vi "Disabled.vi"(7 "Robot Mode":T2, 10 "Match Info":T1={"Autonomous Elapsed Seconds"=0.0, "TeleOp Elapsed Seconds"=0.0, "Disabled Elapsed Seconds"=0.0, "Visited Autonomous"=FALSE, "Visited TeleOp"=FALSE, "Visited Disabled"=FALSE, "Autonomous Settings"={"Autonomous Style"=enum."Independent", "VI Refnum"=refnum}}, 11 "Call Context":T3) -> ()   [LabVIEW 2012]
doc: "This VI is called each time a disabled packet is received from the DS. It is often used to prepare for the next robot mode, to calibrate sensors, etc."
uses:
  <vilib>/Rock Robotics/WPI/DriverStation/WPI_DriverStationDerivedRobotMode.ctl
  <vilib>/Rock Robotics/WPI/DriverStation/WPI_DriverStationRobotMode2.ctl
  <vilib>/Rock Robotics/WPI/DriverStation/WPI_DriverStationMatch Info.ctl
  Robot Global Data.vi
  <vilib>/Rock Robotics/WPI/Joystick/WPI_JoystickGetSetRefNum.vi
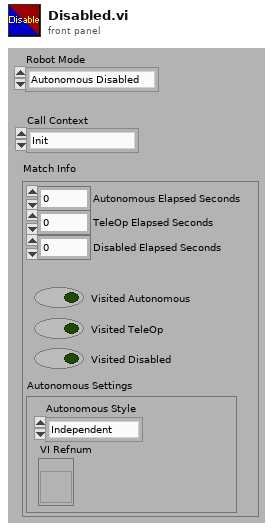
[diagram p1: front panel]
types:
  T1 = typedef "WPI_DriverStationMatch Info.ctl" = cluster{"Autonomous Elapsed Seconds":dbl, "TeleOp Elapsed Seconds":dbl, "Disabled Elapsed Seconds":dbl, "Visited Autonomous":bool, "Visited TeleOp":bool, "Visited Disabled":bool, "Autonomous Settings":cluster{"Autonomous Style":enum16{"Iterative", "Independent"}, "VI Refnum":refnum<vi>}}
  T2 = typedef "WPI_DriverStationRobotMode2.ctl" = enum16{"Autonomous Disabled", "Autonomous Enabled", "Teleop Disabled", "Teleop Enabled", "Timeout", "Finish", "Test Disabled", "Test Enabled"}
  T3 = typedef "WPI_DriverStationDerivedRobotMode.ctl" = enum16{"Init", "Execute", "Stop"}
  T4 = typedef "WPI_JoystickDevRef.ctl" = cluster{"Device":T5}
  T5 = typedef "WPI_JoystickDeviceEnum.ctl" = enum16{"USB 1", "USB 2", "USB 3", "USB 4", "Kinect 1", "Kinect 2"}
  T6 = typedef "WPI_JoystickButtonState.ctl" = cluster{"Button 1":bool, "Button 2":bool, "Button 3":bool, "Button 4":bool, "Button 5":bool, "Button 6":bool, "Button 7":bool, "Button 8":bool, "Button 9":bool, "Button 10":bool, "Button 11":bool, "Button 12":bool}
  T7 = cluster{"FlipperLeftUp":dbl, "FlipperLeftDown":dbl, "FlipperRightUp":dbl, "FlipperRightDown":dbl, "KickerLeftBack":dbl, "KickerLeftForward":dbl, "KickerRightBack":dbl, "KickerRightForward":dbl}
  T8 = typedef "WPI_MotorControlDeviceRef.ctl" = cluster{"DeviceStatus":errorcluster, "Type":enum16{"PWM", "CAN"}, "PWM":cluster{"Digital Module":T9, "PWM Channel":T10, "DeadBand":T11}, "CAN":cluster{"Device Number":u8, "Control Mode":T12, "Semaphore":T13, "Max Vout":dbl}, "Invert":bool, "TransformRef":T14, "InvTransformRef":T14}
  T9 = typedef "FPGA_TypedefDigitalModule.ctl" = enum16{"Digital Module 1", "Digital Module 2"}
  T10 = typedef "FPGA_DIOPWMChannel.ctl" = enum8{"PWM 1", "PWM 2", "PWM 3", "PWM 4", "PWM 5", "PWM 6", "PWM 7", "PWM 8", "PWM 9", "PWM 10", "Invalid"}
  T11 = typedef "WPI_PWMDeadband.ctl" = cluster{"Name":string, "maxPositivePwm":i32, "minPositivePwm":i32, "centerPwm":i32, "maxNegativePwm":i32, "minNegativePwm":i32, "angularRange":u16}
  T12 = typedef "WPI_CANJaguar_ControlMode.ctl" = enum8{"Percent VBus", "Current", "Speed", "Position", "Voltage"}
  T13 = typedef "Semaphore RefNum" = refnum<k1>
  T14 = typedef "WPI_PWMTransform_ConPane.ctl" = refnum<vi>
  T15 = typedef "WPI_ServoDeviceRef.ctl" = cluster{"DeviceStatus":errorcluster, "Digital Module":T9, "PWM Channel":T10, "DeadBand":T11}
  T16 = cluster{"Right Servo High":dbl, "Right Servo Mid":dbl, "Right Servo Low":dbl, "Left Servo High":dbl, "Left Servo Mid":dbl, "Left Servo Low":dbl}
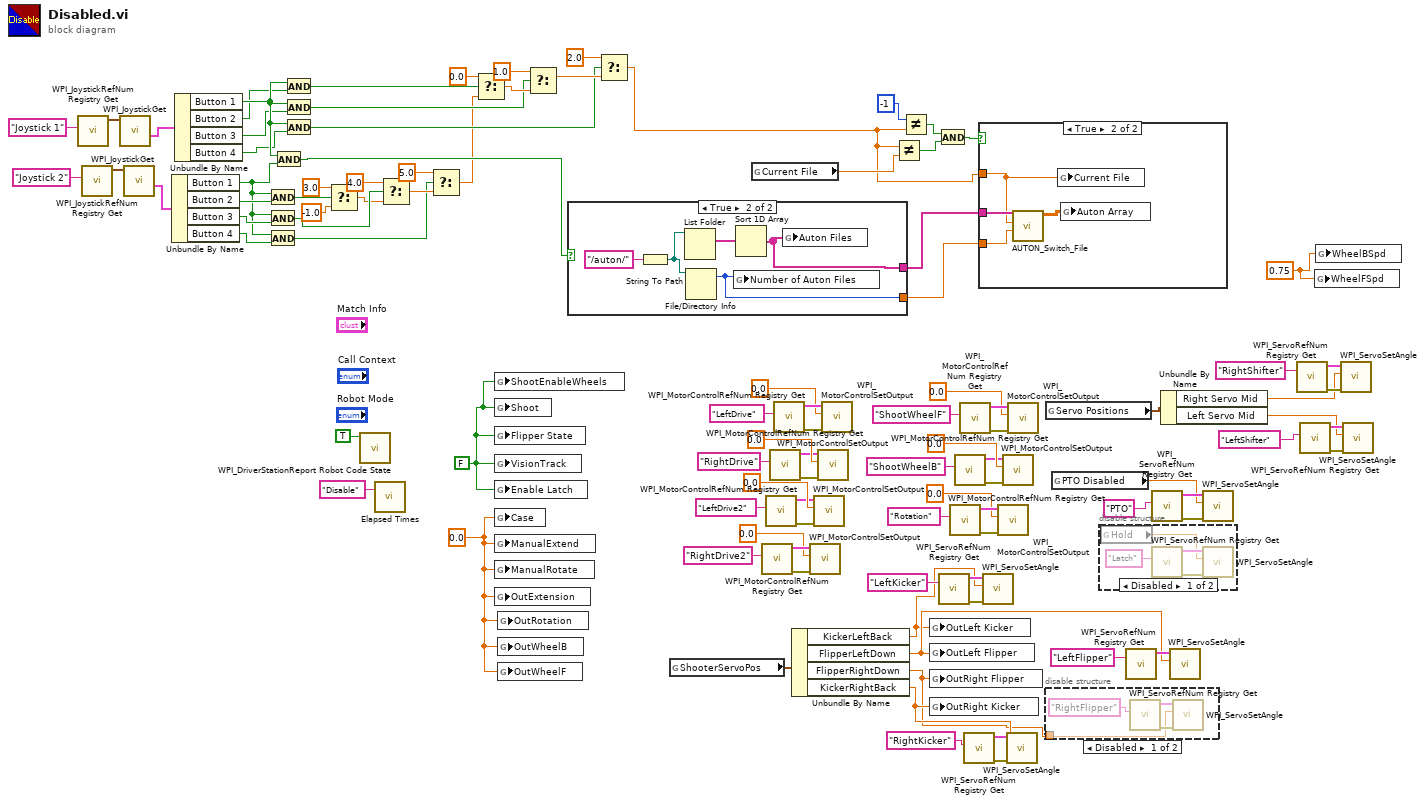
[diagram p0: block diagram]
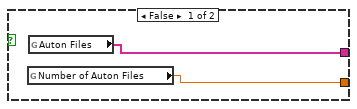
[diagram p5: hidden frame]
diagram:
  w35 = 0.75 ("Case")
  w54 = 0.0 ("Case")
  w55 = FALSE ("Enable Latch")
  n1 = call <vilib>:"WPI_JoystickRefNum Registry Get.vi"("refnum name"="Joystick 1") -> ("JoystickDevRef"=w33:T4)  [unwired: 9 in, 1 out]
  n2 = call <vilib>:"WPI_JoystickRefNum Registry Get.vi"("refnum name"="Joystick 2") -> ("JoystickDevRef"=w31:T4)  [unwired: 9 in, 1 out]
  n3 = call <vilib>:"WPI_JoystickGet.vi"("JoystickDevRef"=w33) -> ("Buttons"=w29:T6)  [unwired: 4 in, 2 out]
  n4 = call <vilib>:"WPI_JoystickGet.vi"("JoystickDevRef"=w31) -> ("Buttons"=w30:T6)  [unwired: 4 in, 2 out]
  n5 = Unbundle By Name(w30) -> ("Button 1"=w26:bool, "Button 2"=w28:bool, "Button 3"=w27:bool, "Button 4"=w25:bool)
  n6 = Unbundle By Name(w29) -> ("Button 1"=w7:bool, "Button 2"=w6:bool, "Button 3"=w5:bool, "Button 4"=w4:bool)
  n7 = And(x=w26, y=w28) -> (x .and. y?=w24:bool)
  n8 = And(x=w26, y=w27) -> (x .and. y?=w21:bool)
  n9 = And(x=w26, y=w25) -> (x .and. y?=w15:bool)
  n10 = And(x=w7, y=w26) -> (x .and. y?=w17:bool)
  n11 = And(x=w7, y=w6) -> (x .and. y?=w8:bool)
  n12 = And(x=w7, y=w5) -> (x .and. y?=w10:bool)
  n13 = And(x=w7, y=w4) -> (x .and. y?=w3:bool)
  n14 = Select(t=3.0, s=w24, f=-1.0) -> (s? t:f=w20:dbl)
  n15 = call <vilib>:"WPI_DriverStationReport Robot Code State.vi"("Disabled"=TRUE ("Autonomous")) -> ()  [unwired: 10 in, 1 out]
  n16 = call "Elapsed Times.vi"("Call Name"="Disable") -> ()  [unwired: 2 in, 1 out]
  n17 = Select(t=4.0, s=w21, f=w20) -> (s? t:f=w18:dbl)
  n18 = Select(t=5.0, s=w15, f=w18) -> (s? t:f=w2:dbl)
  n19 = Select(t=0.0, s=w8, f=w2) -> (s? t:f=w11:dbl)
  n20 = global write "Robot Global Data.vi" "ShootEnableWheels"(w55) -> ()
  n21 = global write "Robot Global Data.vi" "Shoot"(w55) -> ()
  n22 = global write "Robot Global Data.vi" "Flipper State"(w55) -> ()
  n23 = global write "Robot Global Data.vi" "VisionTrack"(w55) -> ()
  n24 = global write "Robot Global Data.vi" "Enable Latch"(w55) -> ()
  n25 = global write "Robot Global Data.vi" "Case"(w54) -> ()
  n26 = global write "Robot Global Data.vi" "ManualExtend"(w54) -> ()
  n27 = global write "Robot Global Data.vi" "ManualRotate"(w54) -> ()
  n28 = global write "Robot Global Data.vi" "OutExtension"(w54) -> ()
  n29 = global write "Robot Global Data.vi" "OutRotation"(w54) -> ()
  n30 = global write "Robot Global Data.vi" "OutWheelB"(w54) -> ()
  n31 = global write "Robot Global Data.vi" "OutWheelF"(w54) -> ()
  n32 = Select(t=1.0, s=w10, f=w11) -> (s? t:f=w13:dbl)
  n33 = case shown="True" w17 {
    tunnel: [w101 w104] -> w90
    tunnel: [w102 w103] -> w85
    frame False {
      n34 = global read "Robot Global Data.vi" "Number of Auton Files"() -> (w101:dbl)
      n35 = global read "Robot Global Data.vi" "Auton Files"() -> (w102:string[])
    }
    frame True {
      n36 = String To Path(string="/auton/") -> (path=w106:path)
      n37 = List Folder(path=w106) -> (filenames=w105:string[])  [unwired: 3 in, 3 out]
      n38 = File/Directory Info(path=w106) -> (size=w104:i64)  [unwired: 1 in, 6 out]
      n39 = global write "Robot Global Data.vi" "Number of Auton Files"(w104) -> ()
      n40 = Sort 1D Array(array=w105) -> (sorted array=w103:string[])
      n41 = global write "Robot Global Data.vi" "Auton Files"(w103) -> ()
    }
  }
  n42 = Select(t=2.0, s=w3, f=w13) -> (s? t:f=w1:dbl)
  n43 = global read "Robot Global Data.vi" "ShooterServoPos"() -> (w53:T7)
  n44 = global read "Robot Global Data.vi" "Current File"() -> (w88:dbl)
  n45 = call <vilib>:"WPI_MotorControlRefNum Registry Get.vi"("refnum name"="RightDrive2") -> ("error out"=w71:errorcluster, "MotorControlDevRef"=w70:T8)  [unwired: 9 in]
  n46 = call <vilib>:"WPI_MotorControlRefNum Registry Get.vi"("refnum name"="LeftDrive2") -> ("error out"=w64:errorcluster, "MotorControlDevRef"=w65:T8)  [unwired: 9 in]
  n47 = call <vilib>:"WPI_MotorControlRefNum Registry Get.vi"("refnum name"="RightDrive") -> ("error out"=w91:errorcluster, "MotorControlDevRef"=w92:T8)  [unwired: 9 in]
  n48 = call <vilib>:"WPI_MotorControlRefNum Registry Get.vi"("refnum name"="LeftDrive") -> ("error out"=w98:errorcluster, "MotorControlDevRef"=w97:T8)  [unwired: 9 in]
  n49 = Unbundle By Name(w53) -> ("KickerLeftBack"=w50:dbl, "FlipperLeftDown"=w51:dbl, "FlipperRightDown"=w49:dbl, "KickerRightBack"=w52:dbl)
  n50 = call <vilib>:"WPI_MotorControlSetOutput.vi"("error in (no error)"=w71, "Output"=0.0, "MotorControlDevRef"=w70) -> ()  [unwired: 6 in, 3 out]
  n51 = call <vilib>:"WPI_MotorControlSetOutput.vi"("error in (no error)"=w64, "Output"=0.0, "MotorControlDevRef"=w65) -> ()  [unwired: 6 in, 3 out]
  n52 = call <vilib>:"WPI_MotorControlSetOutput.vi"("error in (no error)"=w91, "Output"=0.0, "MotorControlDevRef"=w92) -> ()  [unwired: 6 in, 3 out]
  n53 = call <vilib>:"WPI_MotorControlSetOutput.vi"("error in (no error)"=w98, "Output"=0.0, "MotorControlDevRef"=w97) -> ()  [unwired: 6 in, 3 out]
  n54 = Not Equal?(x=w1, y=w88) -> (x != y?=w86:bool)
  n55 = Not Equal?(x=-1, y=w1) -> (x != y?=w87:bool)
  n56 = global write "Robot Global Data.vi" "OutLeft Kicker"(w50) -> ()
  n57 = global write "Robot Global Data.vi" "OutLeft Flipper"(w51) -> ()
  n58 = global write "Robot Global Data.vi" "OutRight Flipper"(w49) -> ()
  n59 = global write "Robot Global Data.vi" "OutRight Kicker"(w52) -> ()
  n60 = And(x=w87, y=w86) -> (x .and. y?=w84:bool)
  n61 = call <vilib>:"WPI_ServoRefNum Registry Get.vi"("refnum name"="LeftKicker") -> ("error out"=w56:errorcluster, "ServoDeviceRef"=w57:T15)  [unwired: 9 in]
  n62 = call <vilib>:"WPI_MotorControlRefNum Registry Get.vi"("refnum name"="Rotation") -> ("error out"=w75:errorcluster, "MotorControlDevRef"=w74:T8)  [unwired: 9 in]
  n63 = call <vilib>:"WPI_MotorControlRefNum Registry Get.vi"("refnum name"="ShootWheelB") -> ("error out"=w76:errorcluster, "MotorControlDevRef"=w77:T8)  [unwired: 9 in]
  n64 = call <vilib>:"WPI_MotorControlRefNum Registry Get.vi"("refnum name"="ShootWheelF") -> ("error out"=w83:errorcluster, "MotorControlDevRef"=w82:T8)  [unwired: 9 in]
  n65 = call <vilib>:"WPI_ServoRefNum Registry Get.vi"("refnum name"="RightKicker") -> ("error out"=w62:errorcluster, "ServoDeviceRef"=w60:T15)  [unwired: 9 in]
  n66 = case shown="True" w84 {
    tunnel: w85 -> [_ w111]
    tunnel: w90 -> [_ w110]
    tunnel: w1 -> [_ w108]
    frame False {
    }
    frame True {
      n67 = call "AUTON_Switch_File.vi"("Number of Auton Files"=w110, "Auton File"=w108, "Auton Files"=w111) -> ("Auton Array"=w109:dbl[][])  [unwired: 7 in, 1 out]
      n68 = global write "Robot Global Data.vi" "Current File"(w108) -> ()
      n69 = global write "Robot Global Data.vi" "Auton Array"(w109) -> ()
    }
  }
  n70 = call <vilib>:"WPI_ServoSetAngle.vi"("error in (no error)"=w56, "Angle"=w50, "ServoDeviceRef"=w57) -> ()  [unwired: 7 in, 2 out]
  n71 = call <vilib>:"WPI_MotorControlSetOutput.vi"("error in (no error)"=w75, "Output"=0.0, "MotorControlDevRef"=w74) -> ()  [unwired: 6 in, 3 out]
  n72 = call <vilib>:"WPI_MotorControlSetOutput.vi"("error in (no error)"=w76, "Output"=0.0, "MotorControlDevRef"=w77) -> ()  [unwired: 6 in, 3 out]
  n73 = call <vilib>:"WPI_ServoSetAngle.vi"("error in (no error)"=w62, "Angle"=w52, "ServoDeviceRef"=w60) -> ()  [unwired: 7 in, 2 out]
  n74 = call <vilib>:"WPI_MotorControlSetOutput.vi"("error in (no error)"=w83, "Output"=0.0, "MotorControlDevRef"=w82) -> ()  [unwired: 6 in, 3 out]
  n75 = global read "Robot Global Data.vi" "Servo Positions"() -> (w39:T16)
  n76 = disable-structure shown="Disabled" {
    disable-tunnel: w49 -> [w112 _]
    frame Disabled {
      n77 = call <vilib>:"WPI_ServoRefNum Registry Get.vi"("refnum name"="RightFlipper") -> ("error out"=w115:errorcluster, "ServoDeviceRef"=w113:T15)  [unwired: 9 in]
      n78 = call <vilib>:"WPI_ServoSetAngle.vi"("error in (no error)"=w115, "Angle"=w112, "ServoDeviceRef"=w113) -> ()  [unwired: 7 in, 2 out]
    }
    frame Enabled {
    }
  }
  n79 = global read "Robot Global Data.vi" "PTO Disabled"() -> (w36:dbl)
  n80 = disable-structure shown="Disabled" {
    frame Disabled {
      n81 = global read "Robot Global Data.vi" "Hold"() -> (w116:dbl)
      n82 = call <vilib>:"WPI_ServoRefNum Registry Get.vi"("refnum name"="Latch") -> ("error out"=w117:errorcluster, "ServoDeviceRef"=w118:T15)  [unwired: 9 in]
      n83 = call <vilib>:"WPI_ServoSetAngle.vi"("error in (no error)"=w117, "Angle"=w116, "ServoDeviceRef"=w118) -> ()  [unwired: 7 in, 2 out]
    }
    frame Enabled {
    }
  }
  n84 = call <vilib>:"WPI_ServoRefNum Registry Get.vi"("refnum name"="LeftFlipper") -> ("ServoDeviceRef"=w58:T15)  [unwired: 9 in, 1 out]
  n85 = call <vilib>:"WPI_ServoRefNum Registry Get.vi"("refnum name"="PTO") -> ("error out"=w40:errorcluster, "ServoDeviceRef"=w42:T15)  [unwired: 9 in]
  n86 = Unbundle By Name(w39) -> ("Right Servo Mid"=w37:dbl, "Left Servo Mid"=w38:dbl)
  n87 = call <vilib>:"WPI_ServoSetAngle.vi"("Angle"=w51, "ServoDeviceRef"=w58) -> ()  [unwired: 8 in, 2 out]
  n88 = call <vilib>:"WPI_ServoSetAngle.vi"("error in (no error)"=w40, "Angle"=w36, "ServoDeviceRef"=w42) -> ()  [unwired: 7 in, 2 out]
  n89 = call <vilib>:"WPI_ServoRefNum Registry Get.vi"("refnum name"="RightShifter") -> ("error out"=w45:errorcluster, "ServoDeviceRef"=w46:T15)  [unwired: 9 in]
  n90 = call <vilib>:"WPI_ServoRefNum Registry Get.vi"("refnum name"="LeftShifter") -> ("error out"=w47:errorcluster, "ServoDeviceRef"=w48:T15)  [unwired: 9 in]
  n91 = global write "Robot Global Data.vi" "WheelFSpd"(w35) -> ()
  n92 = global write "Robot Global Data.vi" "WheelBSpd"(w35) -> ()
  n93 = call <vilib>:"WPI_ServoSetAngle.vi"("error in (no error)"=w45, "Angle"=w37, "ServoDeviceRef"=w46) -> ()  [unwired: 7 in, 2 out]
  n94 = call <vilib>:"WPI_ServoSetAngle.vi"("error in (no error)"=w47, "Angle"=w38, "ServoDeviceRef"=w48) -> ()  [unwired: 7 in, 2 out]
